vi "myRIO_BRig_RT_dataExp_laser2_Power_step.vi"() -> (2 "output_laser2_Power_step":i32)   [LabVIEW 2014]
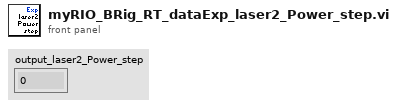
[diagram p1: front panel]
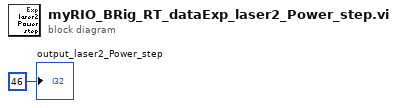
[diagram p0: block diagram]
diagram:
  "output_laser2_Power_step" <- 46 ("output_iBlock")
